vi "Publish Report.vi"(8 "error in (no error)":errorcluster, 11 "Report in":refnum<class "Report.lvclass">) -> (0 "error out":errorcluster, 3 "Report out":refnum<class "Report.lvclass">)   [LabVIEW 2015, in "Report.lvclass"]
doc: "This VI will write the in-memory report to disk."
uses:
  Report.lvclass
  Report.lvclass/Report.ctl
  Report Information/Report Information.lvclass
  Report Formatters/Base Class/Execution/Formatter.lvclass
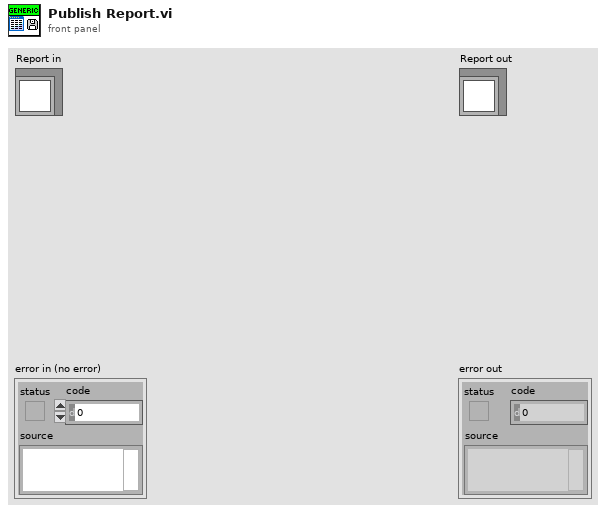
[diagram p1: front panel]
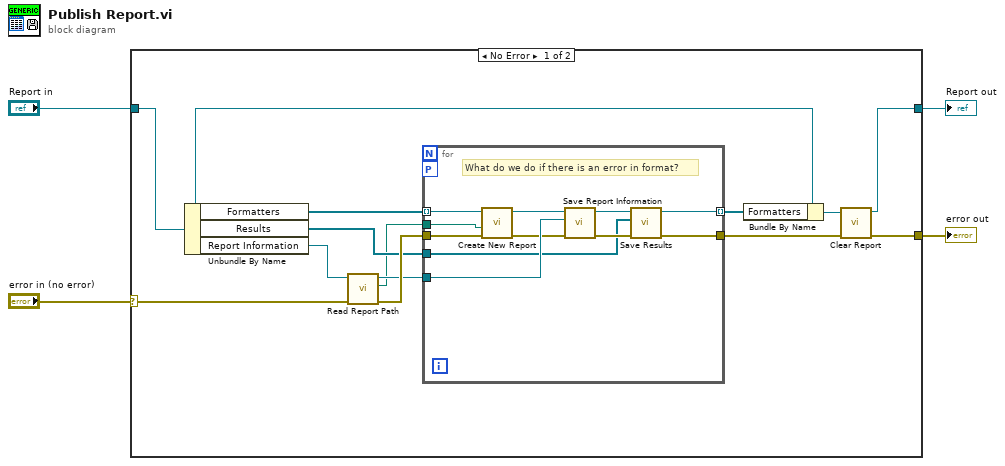
[diagram p0: block diagram]
diagram:
  n1 = case shown="No Error" "error in (no error)" {
    selector: "error in (no error)" -> [w17 w30]
    tunnel: [w8 w30] -> w3
    tunnel: [w5 w29] -> w1
    tunnel: "Report in" -> [w16 w29]
    frame No Error {
      n2 = Unbundle By Name(w16) -> ("Formatters"=w15:refnum<class "Formatter.lvclass">[], "Results"=w10:refnum<class "Result.lvclass">[], "Report Information"=w11:refnum<class "Report Information.lvclass">)
      n3 = call-dynamic "Read Report Path.vi"("error in (no error)"=w17, "Report Information in"=w11) -> ("error out"=w13:errorcluster, "Report Path"=w9:path, "Report Information out"=w12:refnum<class "Report Information.lvclass">)  [unwired: 7 in]
      n4 = for {
        tunnel: w15 -> [w28] mode=indexing
        tunnel: w12 -> [w27]
        tunnel: w10 -> [w23]
        tunnel: [w22] -> w14 mode=indexing
        workers-P: _ -> [_]
        tunnel: w9 -> [w18]
        tunnel: w13 -> [w20]
        tunnel: [w24] -> w7
        # "What do we do if there is an error in format?"
        n5 = call-dynamic "Create New Report.vi"("error in (no error)"=w20, "Report Path"=w18, "Formatter in"=w28) -> ("error out"=w19:errorcluster, "Formatter out"=w21:refnum<class "Formatter.lvclass">)  [unwired: 7 in]
        n6 = call-dynamic "Save Report Information.vi"("error in (no error)"=w19, "Report Information.lvclass"=w27, "Formatter in"=w21) -> ("error out"=w25:errorcluster, "Formatter out"=w26:refnum<class "Formatter.lvclass">)  [unwired: 7 in]
        n7 = call-dynamic "Save Results.vi"("error in (no error)"=w25, "Results"=w23, "Formatter in"=w26) -> ("error out"=w24:errorcluster, "Formatter out"=w22:refnum<class "Formatter.lvclass">)  [unwired: 7 in]
      }
      n8 = Bundle By Name(cluster=w16, "Formatters"=w14) -> (w6:refnum<class "Report.lvclass">)
      n9 = call-dynamic "Clear Report.vi"("error in (no error)"=w7, "Report in"=w6) -> ("error out"=w8:errorcluster, "Report out"=w5:refnum<class "Report.lvclass">)  [unwired: 8 in]
    }
    frame Error {
    }
  }
  "error out" <- w3
  "Report out" <- w1
